vi "saveData.vi"(8 "error in (no error)":errorcluster, 11 "reference in":refnum<class "File Controller.lvclass">) -> (0 "error out":errorcluster, 3 "reference out":refnum<class "File Controller.lvclass">)   [LabVIEW 2015, in "File Controller.lvclass"]
uses:
  File Controller.lvclass
  <vilib>/Utility/config.llb/Write Key (String).vi
  <vilib>/Utility/config.llb/Write Key (Path).vi
  <vilib>/Utility/config.llb/Write Key (Boolean).vi
  <vilib>/Utility/config.llb/NI_LVConfig.lvlib
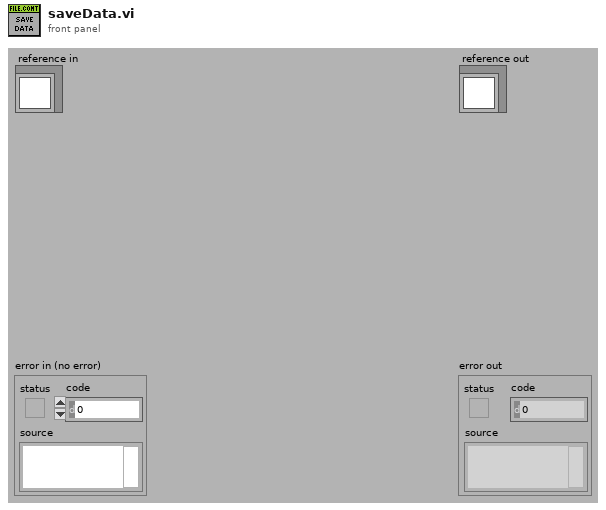
[diagram p1: front panel]
types:
  T1 = typedef "NI_LVConfig.lvlib/Config Data RefNum.ctl" = refnum<k1>
  T2 = typedef "File Controller.lvclass/ObjectAttributesRef.ctl" = refnum<data-value>
  T3 = typedef "File Controller.lvclass/ObjectAttributes.ctl" = cluster{"MyAttribute":dbl, "excelFile_refs":refnum<class "excelFile.lvclass">[], "filePaths":path[], "outlookTemplatePaths":path[], "attachmentTemplatePaths":path[], "configFilePath":path, "not_setting":bool[], "python_ref":refnum<class "python.lvclass">}
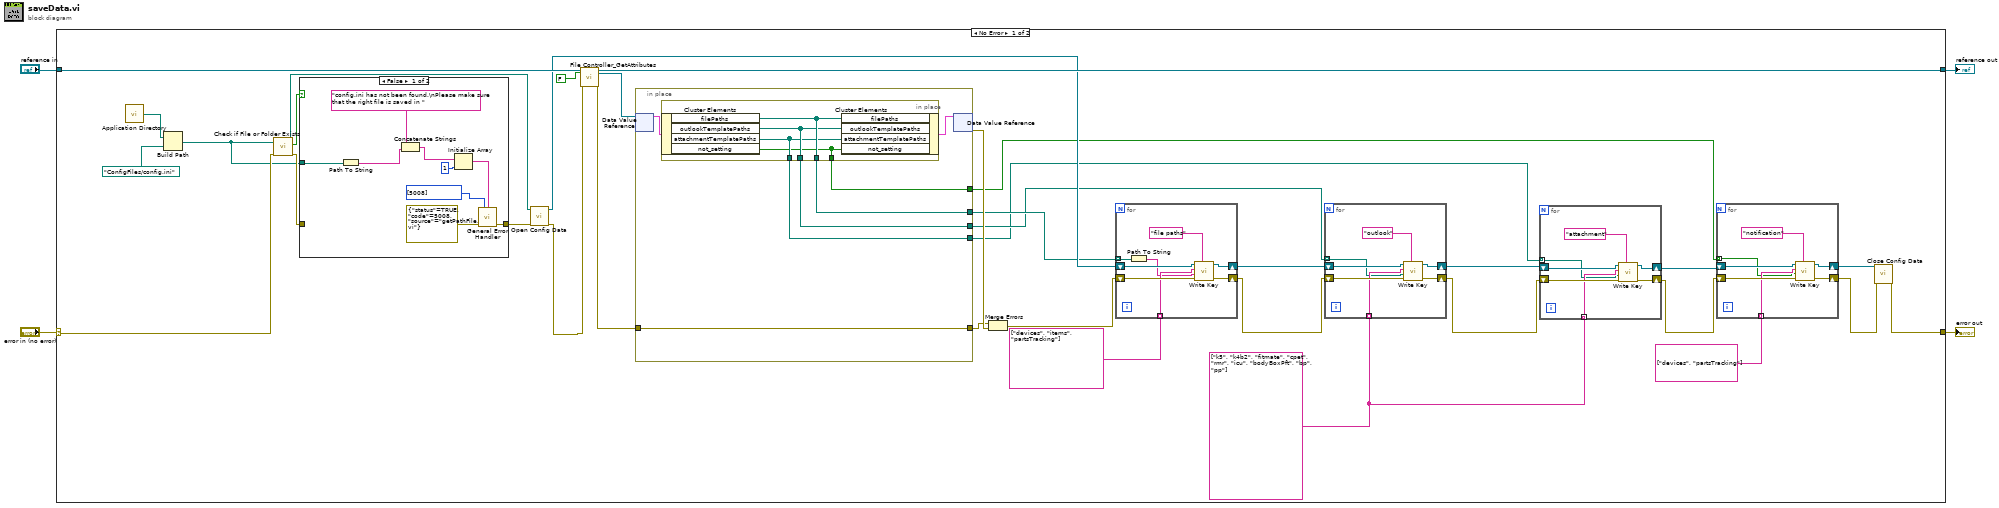
[diagram p0: block diagram]
diagram:
  n1 = case shown="No Error" "error in (no error)" {
    selector: "error in (no error)" -> [w27 w90]
    tunnel: [w14 w90] -> w3
    tunnel: [w33 w89] -> w1
    tunnel: "reference in" -> [w36 w89]
    frame No Error {
      w17 = string[] ["k5", "k4b2", "fitmate", "cpet", "rmr", "icu", "bodyBoxPft", "bp", "pp"]
      n2 = call <vilib>:"Application Directory.vi"() -> ("Application Directory"=w12:path)
      n3 = Build Path(base path=w12, name or relative path=path "ConfigFiles/config.ini" ("path")) -> (appended path=w11:path)
      n4 = call <vilib>:"Check if File or Folder Exists.vi"("error in (no error)"=w27, "path"=w11) -> ("error out"=w31:errorcluster, "file or folder exists?"=w30:bool, "dup path"=w28:path)  [unwired: 7 in]
      n5 = case shown="False" w30 {
        tunnel: w31 -> [_ w77]
        tunnel: [w76 w77] -> w29
        tunnel: w11 -> [w71 _]
        frame False {
          n6 = Path To String(path=w71) -> (string=w73:string)
          n7 = Concatenate Strings("config.ini has not been found.\nPlease make sure that the right file is saved in ", w73) -> (w69:string)
          n8 = Initialize Array(w69, 1 ("dimension size")) -> (w68:string[])
          n9 = call <vilib>:"General Error Handler.vi"("[user-defined codes]"=i32[] [5008], "[user-defined descriptions]"=w68, "error in (no error)"=errorcluster {"status"=TRUE, "code"=5008, "source"="getPathFile.vi"}) -> ("error out"=w76:errorcluster)  [unwired: 8 in, 4 out]
        }
        frame True {
        }
      }
      n10 = call <vilib>:"Open Config Data.vi"("error in (no error)"=w29, "configuration file path"=w28) -> ("error out"=w26:errorcluster, "refnum"=w23:T1)  [unwired: 7 in, 1 out]
      n11 = call "File Controller_GetAttributes.vi"("reference in"=w36, "return data? (T)"=FALSE, "error in (no error)"=w26) -> ("reference out"=w33:refnum<class "File Controller.lvclass">, "attributes ref"=w32:T2, "error out"=w34:errorcluster)  [unwired: 13 in, 1 out]
      n12 = in-place {
        in-place-border: w34 -> [w82]
        in-place-border: [w82] -> w37
        in-place-border: [w81] -> w22
        in-place-border: [w80] -> w19
        in-place-border: [w79] -> w16
        in-place-border: [w78] -> w7
        n13 = in-place-dvr #1(w32) -> (w83:T3)  [unwired: 1 out]
        n14 = in-place {
          in-place-border: [w88] -> w81
          in-place-border: [w87] -> w80
          in-place-border: [w86] -> w79
          in-place-border: [w85] -> w78
          n15 = in-place-cluster #2(w83) -> ("filePaths"=w88:path[], "outlookTemplatePaths"=w87:path[], "attachmentTemplatePaths"=w86:path[], "not_setting"=w85:bool[])
          n16 = in-place-cluster #2("filePaths"=w88, "outlookTemplatePaths"=w87, "attachmentTemplatePaths"=w86, "not_setting"=w85) -> (w84:T3)
        }
        n17 = in-place-dvr #1(w84) -> (w38:errorcluster)  [unwired: 1 out]
      }
      n18 = Merge Errors(w37, w38) -> (w24:errorcluster)
      n19 = for {
        shift-right: [w64] -> w20
        shift-left: w23 -> [w67]
        shift-right: [w63] -> w21
        shift-left: w24 -> [w66]
        tunnel: string[] ["devices", "items", "partsTracking"] -> [w62] mode=indexing
        tunnel: w22 -> [w61] mode=indexing
        n20 = Path To String(path=w61) -> (string=w60:string)
        n21 = call-poly <vilib>:"Write Key.vi"("section"="file paths", "error in (no error)"=w66, "value"=w60, "key"=w62, "refnum"=w67) -> ("error out"=w63:errorcluster, "refnum out"=w64:T1)  [unwired: 4 in, 1 out]
      }
      n22 = for {
        shift-right: [w56] -> w15
        shift-left: w20 -> [w59]
        shift-right: [w55] -> w18
        shift-left: w21 -> [w58]
        tunnel: w17 -> [w54] mode=indexing
        tunnel: w19 -> [w53] mode=indexing
        n23 = call-poly <vilib>:"Write Key.vi"("section"="outlook", "error in (no error)"=w58, "value"=w53, "key"=w54, "refnum"=w59) -> ("error out"=w55:errorcluster, "refnum out"=w56:T1)  [unwired: 4 in, 1 out]
      }
      n24 = for {
        shift-right: [w49] -> w10
        shift-left: w15 -> [w52]
        shift-right: [w48] -> w9
        shift-left: w18 -> [w51]
        tunnel: w17 -> [w47] mode=indexing
        tunnel: w16 -> [w46] mode=indexing
        n25 = call-poly <vilib>:"Write Key.vi"("section"="attachment", "error in (no error)"=w51, "value"=w46, "key"=w47, "refnum"=w52) -> ("error out"=w48:errorcluster, "refnum out"=w49:T1)  [unwired: 4 in, 1 out]
      }
      n26 = for {
        shift-right: [w42] -> w5
        shift-left: w10 -> [w45]
        shift-right: [w41] -> w8
        shift-left: w9 -> [w44]
        tunnel: string[] ["devices", "partsTracking"] -> [w40] mode=indexing
        tunnel: w7 -> [w39] mode=indexing
        n27 = call-poly <vilib>:"Write Key.vi"("section"="notification", "error in (no error)"=w44, "value"=w39, "key"=w40, "refnum"=w45) -> ("error out"=w41:errorcluster, "refnum out"=w42:T1)  [unwired: 4 in, 1 out]
      }
      n28 = call <vilib>:"Close Config Data.vi"("error in (no error)"=w8, "refnum"=w5) -> ("error out"=w14:errorcluster)  [unwired: 8 in, 1 out]
    }
    frame Error {
    }
  }
  "error out" <- w3
  "reference out" <- w1
